vi "InitAttackMap.vi"(1 "Column":i32, 2 "Row":i32) -> (0 "AttackMap DVR":T1)   [LabVIEW 2017, in "Atom.lvclass"]
uses:
  Atom.lvclass
  AttackMap DVR.ctl
  Common/Position.ctl
  SubVIs/Read-Only Globals.vi
  SubVIs/Globals (private).vi
  Square/Square.lvclass
  Common/Common.lvlib
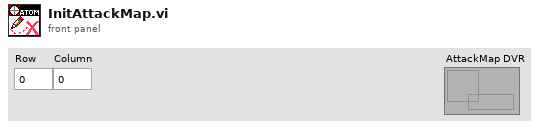
[diagram p1: front panel]
types:
  T1 = typedef "Atom.lvclass/AttackMap DVR.ctl" = refnum<data-value>
  T2 = typedef "Common.lvlib/Position.ctl" = cluster{"Column":i32, "Row":i32}
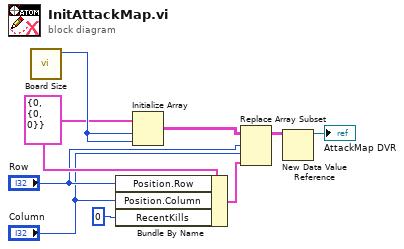
[diagram p0: block diagram]
diagram:
  w5 = cluster{"RecentKills":i32, "Position":T2} {"RecentKills"=0, "Position"={"Column"=0, "Row"=0}} ("new element/subarray")
  n1 = call "Board Size.vi"() -> ("Board Size"=w7:i32)  [unwired: 11 in]
  n2 = Bundle By Name(cluster=w5, "Position.Row"="Row", "Position.Column"="Column", "RecentKills"=0) -> (w4:cluster{"RecentKills":i32, "Position":T2})
  n3 = Initialize Array(w5, w7, w7) -> (w6:cluster{"RecentKills":i32, "Position":T2}[][])
  n4 = Replace Array Subset(array=w6, new element=w4, index (row)="Row", index (col)="Column") -> (w9:cluster{"RecentKills":i32, "Position":T2}[][])
  n5 = New Data Value Reference(data value=w9) -> (data value reference=→"AttackMap DVR":refnum<data-value>)  [unwired: 1 in, 1 out]
